vi "SingleWire_drift_correction_PN.vi"(0 "calib consts. t1":dbl[](array[numeric]), 1 "Tmeas (degC)":dbl, 2 "variable n":bool, 5 "calib consts. t2":dbl[](array[numeric]), 7 "{E_cal1}":dbl[](array[numeric]), 9 "{U_cal1}":dbl[](array[numeric]), 11 "time fraction":dbl, 12 "wire diameter (mu.m)":dbl=5.0) -> (4 "[A, B, n]":dbl[](array[numeric]))   [LabVIEW 2011]
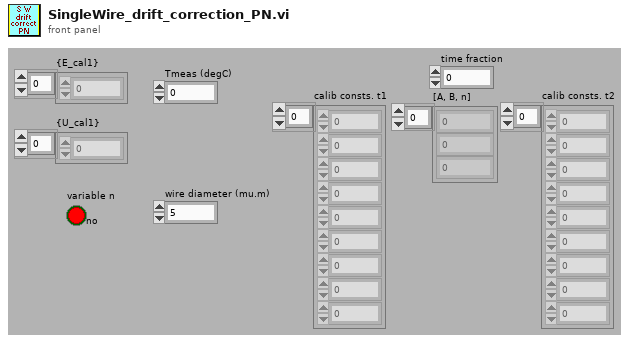
[diagram p1: front panel]
types:
  T1 = cluster{"calib consts. t1[0]":dbl, "calib consts. t1[1]":dbl, "calib consts. t1[2]":dbl, "calib consts. t1[3]":dbl, "calib consts. t1[4]":dbl, "calib consts. t1[5]":dbl, "calib consts. t1[6]":dbl, "calib consts. t1[7]":dbl}
  T2 = cluster{"calib consts. t2[0]":dbl, "calib consts. t2[1]":dbl, "calib consts. t2[2]":dbl, "calib consts. t2[3]":dbl, "calib consts. t2[4]":dbl, "calib consts. t2[5]":dbl, "calib consts. t2[6]":dbl, "calib consts. t2[7]":dbl}
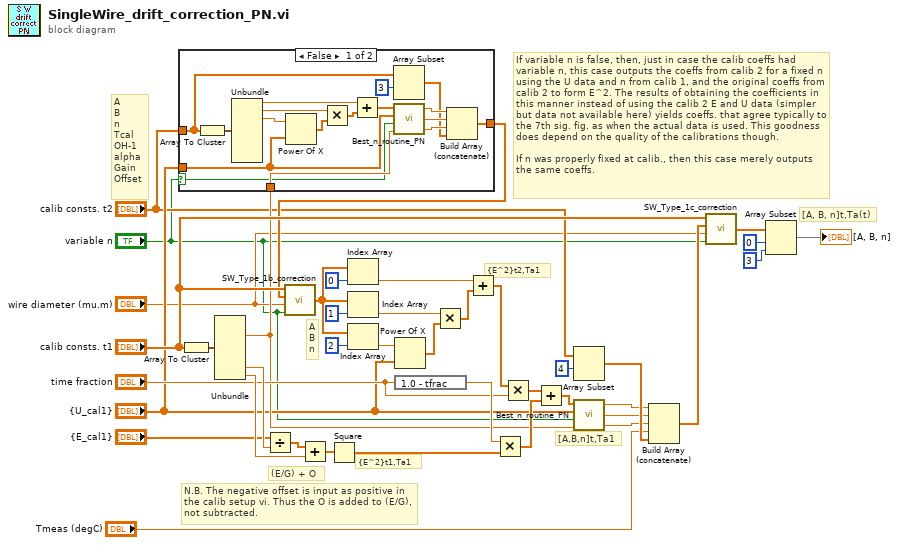
[diagram p0: block diagram]
diagram:
  # "If variable n is false, then, just in case the calib coeffs had variable n, this case outputs the coeffs from calib 2 for a fixed n using the U data and n from calib 1, and the original coeffs from calib 2 to form E^2. The results of obtaining the coefficients in this manner instead of using the calib 2 E and U data (simpler but data not available here) yields coeffs. that agree typically to the 7th sig. fig. as when the actual data is used. This goodness does depend on the quality of the calibrations though.\n\nIf n was properly fixed at calib., then this case merely outputs the same coeffs."
  # "[A, B, n]t,Ta(t)"
  # "[A,B,n]t,Ta1"
  # "{E^2}t2,Ta1"
  # "A\nB\nn"
  # "{E^2}t1,Ta1"
  # "N.B. The negative offset is input as positive in the calib setup vi. Thus the O is added to (E/G), not subtracted."
  # "(E/G) + O"
  # "A\nB\nn\nTcal\nOH-1\nalpha\nGain\nOffset"
  n1 = Array To Cluster(array="calib consts. t1") -> (cluster=w39:T1)
  n2 = Unbundle(w39) -> ("calib consts. t1[2]"=w6:dbl, "calib consts. t1[6]"=w37:dbl, "calib consts. t1[7]"=w38:dbl)  [unwired: 5 out]
  n3 = case shown="False" "variable n" {
    selector: "variable n" -> [w42 _]
    tunnel: w6 -> [w51 _]
    tunnel: "{U_cal1}" -> [w50 _]
    tunnel: [w44 w58] -> w4
    tunnel: "calib consts. t2" -> [w43 w58]
    frame False {
      n4 = Array To Cluster(array=w43) -> (cluster=w57:T2)
      n5 = Unbundle(w57) -> ("calib consts. t2[0]"=w54:dbl, "calib consts. t2[1]"=w53:dbl, "calib consts. t2[2]"=w41:dbl)  [unwired: 5 out]
      n6 = Power Of X(1:w50, 2:w41) -> (0:w56:dbl[])
      n7 = Multiply(x=w53, y=w56) -> (x*y=w55:dbl[])
      n8 = Add(x=w54, y=w55) -> (x+y=w52:dbl[])
      n9 = Array Subset(array=w43, index=3) -> (w45:dbl[])  [unwired: 1 in]
      n10 = call "Best_n_routine_PN.vi"("fixed n"=w51, "variable n?"=w42, "U"=w50, "E^2"=w52) -> ("n"=w46:dbl, "B"=w47:dbl, "A"=w48:dbl)
      n11 = Build Array (concatenate)(w48, w47, w46, w45) -> (w44:dbl[])
    }
    frame True {
    }
  }
  n12 = Divide(x="{E_cal1}", y=w37) -> (x/y=w40:dbl[])
  n13 = call "SW_Type_1b_correction.vi"("variable n"="variable n", "wire diameter (mu.m)"="wire diameter (mu.m)", "calib consts. t2"=w4, "calib consts. t1"="calib consts. t1") -> ("Corrected calib consts. t2"=w34:dbl[])
  n14 = Add(x=w40, y=w38) -> (x+y=w36:dbl[])
  n15 = Square(x=w36) -> (x^2=w26:dbl[])
  n16 = Index Array(array=w34, index=0) -> (element=w30:dbl)
  n17 = Index Array(array=w34, index=1) -> (element=w29:dbl)
  n18 = Index Array(array=w34, index=2) -> (element=w7:dbl)
  n19 = Power Of X(1:"{U_cal1}", 2:w7) -> (0:w27:dbl[])
  n20 = expression code="1.0 - tfrac"("time fraction") -> (w25:dbl)
  n21 = Multiply(x=w29, y=w27) -> (x*y=w28:dbl[])
  n22 = Add(x=w30, y=w28) -> (x+y=w23:dbl[])
  n23 = Multiply(x=w25, y=w26) -> (x*y=w21:dbl[])
  n24 = Multiply(x=w23, y="time fraction") -> (x*y=w22:dbl[])
  n25 = Add(x=w22, y=w21) -> (x+y=w20:dbl[])
  n26 = Array Subset(array="calib consts. t2", index=4) -> (w13:dbl[])  [unwired: 1 in]
  n27 = call "Best_n_routine_PN.vi"("fixed n"=w6, "variable n?"="variable n", "U"="{U_cal1}", "E^2"=w20) -> ("n"=w10:dbl, "B"=w11:dbl, "A"=w12:dbl)
  n28 = Build Array (concatenate)(w12, w11, w10, "Tmeas (degC)", w13) -> (w8:dbl[])
  n29 = call "SW_Type_1c_correction.vi"("variable n"="variable n", "wire diameter (mu.m)"="wire diameter (mu.m)", "calib consts. t"=w8, "calib consts. t1"="calib consts. t1") -> ("Corrected calib consts. t"=w19:dbl[])
  n30 = Array Subset(array=w19, index=0, length=3) -> (→"[A, B, n]":dbl[])
